vi "Write Pic Height.vi"(8 "error in":errorcluster, 10 "Pic Height":i16, 11 "Popup in":refnum<class "Popup.lvclass">) -> (0 "error out":errorcluster, 3 "Popup out":refnum<class "Popup.lvclass">)   [LabVIEW 2021, in "Pop-Up.lvlib" / "Popup.lvclass"]
doc: "Write the custom picture height\n\n<b>Code Developed By:</b>\nTechnology Service Corporation\n1983 S Liberty Drive\nBloomington, IN 47403\nPhone: 812 558-7100\nwww.tsc.com/atcs\n\nDeveloper:\nDaniel Coons"
uses:
  Popup.lvclass
  Popup.lvclass/Popup.ctl
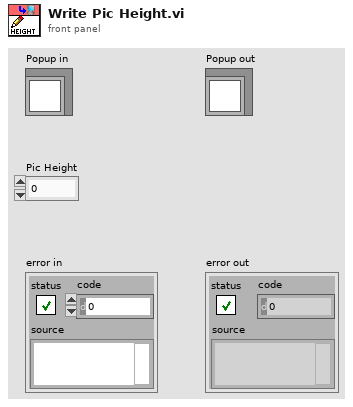
[diagram p1: front panel]
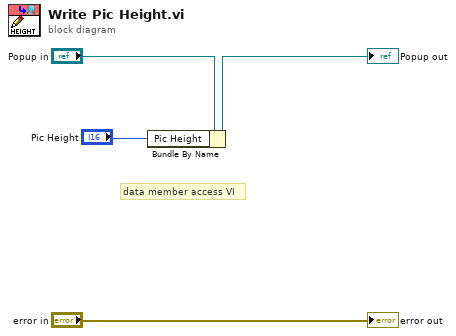
[diagram p0: block diagram]
diagram:
  # "data member access VI"
  n1 = Bundle By Name(cluster="Popup in", "Pic Height"="Pic Height") -> (→"Popup out":refnum<class "Popup.lvclass">)
  "error out" <- "error in"
